vi "TangoAttributeConfigEventTest.vi"() -> ()   [LabVIEW 2014, in "examples.lvlib"]
uses:
  examples.lvlib
  vis/tango_vi.llb/tango.lvlib
panel:
  out "Attr: double_scalar":T1
  out "Attr: long_scalar":T1
  out "?":string="\n1. Be sure your TangoTest device is running \n\n2. Open Jive in read/write mode\n\n3. Click on the 'Device' tab \n\n4. Locate your TangoTest device in the devices tree\n\n5. Expand  the corresponding entry \n\n6. Click on 'Attribute config'\n\n7. Change any component of the configuration of the'long_scalar' or 'double_scalar' attribute\n\n8. This LabVIEW example should receive a notification of your atrribute configuration modification"
  in  "?":bool
  in  "TangoTest Device Name":string="sys/tg_test/1"
  # "TANGO \"ATTRIBUTE CONFIG CHANGED\" EVENT DEMO"
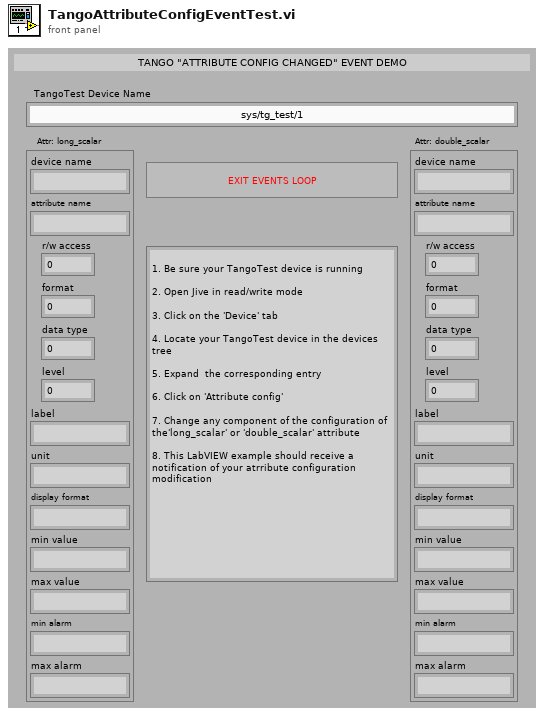
[diagram p1: front panel]
types:
  T1 = cluster{"device name":string, "attribute name":string, "r/w access":i16, "format":i16, "data type":i16, "level":i16, "label":string, "unit":string, "display format":string, "min value":string, "max value":string, "min alarm":string, "max alarm":string}
  T2 = typedef "tango.lvlib/_AttributeConfigEventRef.ctl" = cluster{"attribute info":refnum<user-event>, "Event Registration Refnum":refnum<event-registration>}
  T3 = typedef "tango.lvlib/_AttributeInfo_t.ctl" = cluster{"device name":string, "attribute name":string, "r/w access":T4, "format":T5, "data type":T6, "level":T7, "label":string, "unit":string, "display format":string, "min value":string, "max value":string, "min alarm":string, "max alarm":string}
  T4 = typedef "tango.lvlib/_AttributeAccess_t.ctl" = enum16{"READ", "READ_WITH_WRITE", "WRITE", "READ_WRITE", "UNKNOWN_ACCESS_TYPE"}
  T5 = typedef "tango.lvlib/_AttributeFormat_t.ctl" = enum16{"SCALAR", "SPECTRUM", "IMAGE", "UNKNOWN_FORMAT"}
  T6 = typedef "tango.lvlib/_TangoDataType_t.ctl" = enum16{"VOID", "BOOLEAN", "SHORT", "LONG", "FLOAT", "DOUBLE", "USHORT", "ULONG", "STRING", "CHAR_ARRAY", "SHORT_ARRAY", "LONG_ARRAY", "FLOAT_ARRAY", "DOUBLE_ARRAY", "USHORT_ARRAY", "ULONG_ARRAY", "STRING_ARRAY", "LONG_STRING_ARRAY", "DOUBLE_STRING_ARRAY", "STATE", "CONST_STRING", "BOOLEAN_ARRAY", "UCHAR", "LONG64", "ULONG64", "LONG64_ARRAY", "ULONG64_ARRAY", "INT (not supported)", "ENCODED (not supported)", "ENUM", "PIPE_BLOB (not supported)", "STATE_ARRAY", "UNKNOW_DATA_TYPE"}
  T7 = typedef "tango.lvlib/_AttributeLevel_t.ctl" = enum16{"OPERATOR", "EXPERT", "UNKNOWN_LEVEL"}
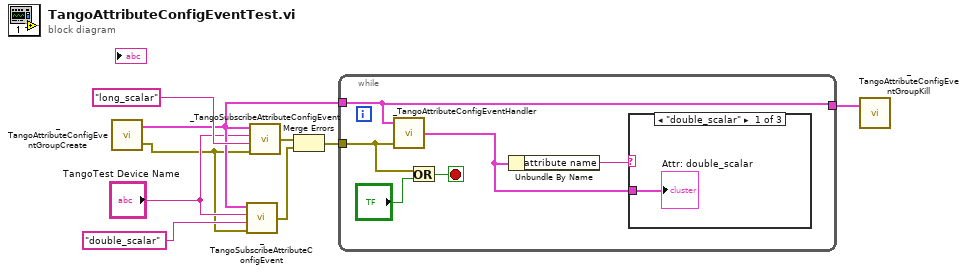
[diagram p0: block diagram]
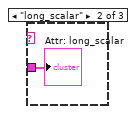
[diagram p2: hidden frame]
diagram:
  n1 = call "_TangoAttributeConfigEventGroupCreate.vi"() -> ("attribute config event ref"=w7:T2, "error out"=w4:errorcluster)  [unwired: 1 in]
  n2 = call "_TangoSubscribeAttributeConfigEvent.vi"("error in"=w4, "attribute name"="double_scalar", "device name"="TangoTest Device Name", "attribute config event ref"=w7) -> ("error out"=w2:errorcluster)
  n3 = call "_TangoSubscribeAttributeConfigEvent.vi"("error in"=w4, "attribute name"="long_scalar", "device name"="TangoTest Device Name", "attribute config event ref"=w7) -> ("error out"=w3:errorcluster)
  n4 = Merge Errors(w3, w2) -> (w1:errorcluster)
  n5 = while {
    tunnel: w7 -> [w10]
    tunnel: w1 -> [w13]
    tunnel: [w10] -> w8
    stop <- w11 stop-if-true
    n6 = call "_TangoAttributeConfigEventHandler.vi"("error in"=w13, "attribute config event ref"=w10) -> ("attribute info"=w14:T3)  [unwired: 1 in, 2 out]
    n7 = Or(x=w13, y="?") -> (x .or. y?=w11:bool)
    n8 = Unbundle By Name(w14) -> ("attribute name"=w15:string)
    n9 = case shown="\"double_scalar\"" w15 {
      tunnel: w14 -> [w16 w17 _]
      frame "double_scalar" {
        "Attr: double_scalar" <- w16
      }
      frame "long_scalar" {
        "Attr: long_scalar" <- w17
      }
      frame Default {
      }
    }
  }
  n10 = call "_TangoAttributeConfigEventGroupKill.vi"("attribute config event ref"=w8) -> ()  [unwired: 1 in, 1 out]
